vi "Periodic Tasks.vi"(8 "error in":errorcluster) -> ()   [LabVIEW 2018]
doc: "This VI runs in parallel to other tasks. It can contain as many user-defined periodic loops as you need. These can carry out PID or other sorts of timed response."
uses:
  <vilib>/Rock Robotics/WPI/ThirdParty/Sensors/navX/_TypeDefs/FRIC_navX_DeviceNumbersTypeDef.ctl
  <vilib>/Rock Robotics/WPI/DriverStation/WPI_DriverStationDerivedRobotMode.ctl
  <vilib>/Rock Robotics/WPI/DriverStation/WPI_DriverStationRobotMode2.ctl
  <vilib>/Rock Robotics/WPI/ThirdParty/Sensors/navX/_Processing Loop/FRIC_navX_Internal_SPI_ProcessingLoop.vi
  Robot Global Data.vi
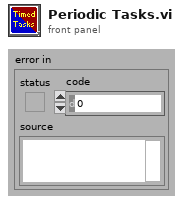
[diagram p1: front panel]
types:
  T1 = typedef "FRIC_navX_DeviceNumbersTypeDef.ctl" = enum16{"Dev0", "Dev1", "Dev2", "Dev3"}
  T2 = typedef "WPI_DriverStationRobotMode2.ctl" = enum16{"Autonomous Disabled", "Autonomous Enabled", "Teleop Disabled", "Teleop Enabled", "Disconnected", "Finish", "Test Disabled", "Test Enabled", "Emergency Stopped"}
  T3 = typedef "WPI_DriverStationDerivedRobotMode.ctl" = enum16{"Init", "Execute", "Stop"}
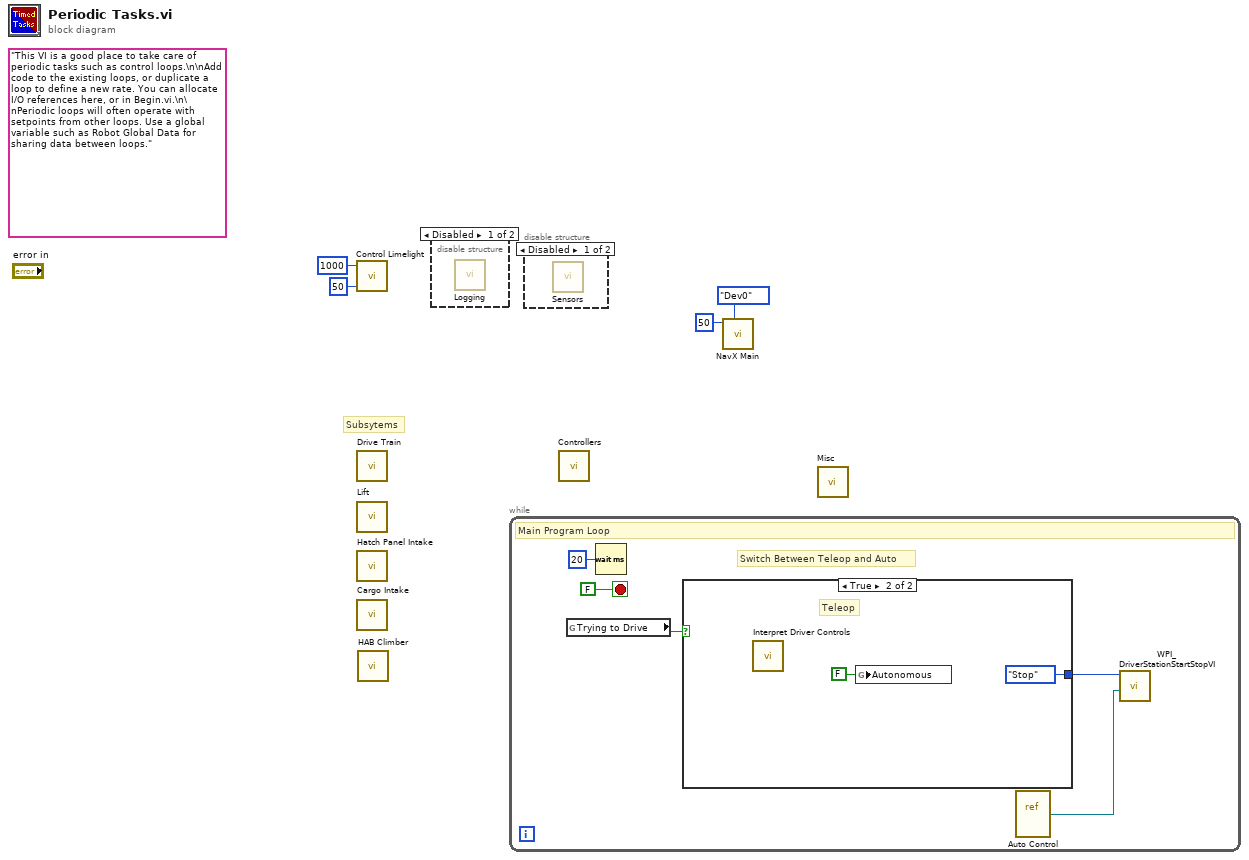
[diagram p0: block diagram]
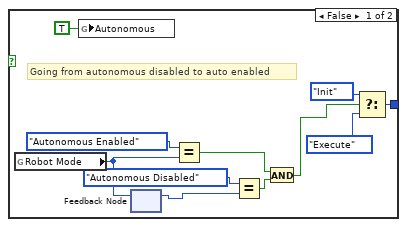
[diagram p2: hidden frame]
diagram:
  (unwired) "This VI is a good place to take care of periodic tasks such as control loops.\n\nAdd code to the existing loops, or duplicate a loop to define a new rate. You can allocate I/O references here, or in Begin.vi.\n\nPeriodic loops will often operate with setpoints from other loops. Use a global variable such as Robot Global Data for sharing data between loops."
  # "Subsytems"
  n1 = call "Control Limelight.vi"("Read Data Loop Time (ms) (min 10)"=u32 50, "Write Data Loop Time (ms)"=u32 1000) -> ()  [unwired: 1 in]
  n2 = call "Drive Train.vi"() -> ()  [unwired: 12 in]
  n3 = call "Lift.vi"() -> ()  [unwired: 1 in]
  n4 = call "Hatch Panel Intake.vi"() -> ()  [unwired: 10 in]
  n5 = call "Cargo Intake.vi"() -> ()  [unwired: 12 in]
  n6 = call "HAB Climber.vi"() -> ()  [unwired: 12 in]
  n7 = disable-structure shown="Disabled" {
    frame Disabled {
      n8 = call "Logging.vi"() -> ()  [unwired: 12 in]
    }
    frame Enabled {
    }
  }
  n9 = while {
    stop <- FALSE stop-if-true
    # "Switch Between Teleop and Auto"
    # "Main Program Loop"
    n10 = global read "Robot Global Data.vi" "Trying to Drive"() -> (w7:bool)
    n11 = Wait (ms)(milliseconds to wait=u32 20) -> ()  [unwired: 1 out]
    n12 = case shown="True" w7 {
      tunnel: [w19 WPI_DriverStationDerivedRobotMode."Stop" ("f")] -> w6
      frame False {
        # "Going from autonomous disabled to auto enabled"
        n13 = global read "Robot Global Data.vi" "Robot Mode"() -> (w16:T2)
        n14 = global write "Robot Global Data.vi" "Autonomous"(TRUE ("Autonomous")) -> ()
        n15 = feedback #1() -> (w13:T2)  [unwired: 1 in]
        n16 = feedback-in #1(w16) -> ()
        n17 = Equal?(x=WPI_DriverStationRobotMode2."Autonomous Enabled" ("y"), y=w16) -> (x = y?=w11:bool)
        n18 = Equal?(x=WPI_DriverStationRobotMode2."Autonomous Disabled" ("y"), y=w13) -> (x = y?=w12:bool)
        n19 = And(x=w11, y=w12) -> (x .and. y?=w10:bool)
        n20 = Select(t=WPI_DriverStationDerivedRobotMode."Init" ("Call Context"), s=w10, f=WPI_DriverStationDerivedRobotMode."Execute") -> (s? t:f=w19:T3)
      }
      frame True {
        # "Teleop"
        n21 = call "Interpret Driver Controls.vi"() -> ()  [unwired: 12 in]
        n22 = global write "Robot Global Data.vi" "Autonomous"(FALSE ("Autonomous")) -> ()
      }
    }
    n23 = vi-ref "Auto Control.vi"() -> (w5:refnum<vi>)
    n24 = call <vilib>:"WPI_DriverStationStartStopVI.vi"("VI in"=w5, "Call Context"=w6) -> ()  [unwired: 10 in]
  }
  n25 = disable-structure shown="Disabled" {
    frame Disabled {
      n26 = call "Sensors.vi"() -> ()  [unwired: 12 in]
    }
    frame Enabled {
    }
  }
  n27 = call "Controllers.vi"() -> ()  [unwired: 12 in]
  n28 = call-poly <vilib>:"NavX Main.vi"("Device Number"=FRIC_navX_DeviceNumbersTypeDef."Dev0", "Rate (4Hz-200Hz)"=u8 50) -> ()  [unwired: 10 in]
  n29 = call "Misc.vi"() -> ()  [unwired: 12 in]
